vi "copy_to_network_and_server.vi"(11 "Path":path) -> ()   [LabVIEW 2016]
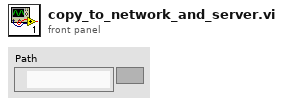
[diagram p1: front panel]
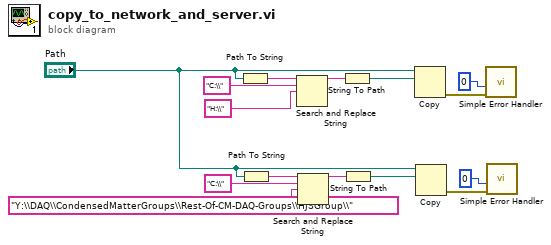
[diagram p0: block diagram]
diagram:
  n1 = Path To String(path="Path") -> (string=w3:string)
  n2 = Path To String(path="Path") -> (string=w8:string)
  n3 = Search and Replace String(input string=w3, search string="C:\\", replace string="H:\\") -> (result string=w1:string)  [unwired: 5 in, 3 out]
  n4 = Search and Replace String(input string=w8, search string="C:\\", replace string="Y:\\DAQ\\CondensedMatterGroups\\Rest-Of-CM-DAQ-Groups\\HJSGroup\\") -> (result string=w6:string)  [unwired: 5 in, 3 out]
  n5 = String To Path(string=w1) -> (path=w2:path)
  n6 = String To Path(string=w6) -> (path=w7:path)
  n7 = Copy(10:w2, 11:"Path") -> (0:w13:errorcluster)  [unwired: 3 in, 2 out]
  n8 = Copy(10:w7, 11:"Path") -> (0:w15:errorcluster)  [unwired: 3 in, 2 out]
  n9 = call <vilib>:"Simple Error Handler.vi"("type of dialog (OK msg:1)"=0, "error in (no error)"=w13) -> ()  [unwired: 3 in, 5 out]
  n10 = call <vilib>:"Simple Error Handler.vi"("type of dialog (OK msg:1)"=0, "error in (no error)"=w15) -> ()  [unwired: 3 in, 5 out]
